vi "SW_Select_User.vi"() -> ()   [LabVIEW 2016]
uses:
  <vilib>/Utility/miscctls.llb/LVPointTypeDef.ctl
  <vilib>/Utility/config.llb/NI_LVConfig.lvlib
panel:
  out "TestComm indicator for Latching inside Events workaround":bool
  in  "Login tab":enum32{"Login", "Settings", "Manage users"}(tab)
  in  "Go to Tracker":bool
  in  "Select User":u16(ring) items=["Admin"]
  in  "Enter password":string
  in  "Jump to tracking":bool
  out "Comm. test results":bool
  in  "Test VISA Comms":bool
  in  "Save Settings":bool
  in  "VISA":refnum<visa-resource-name>="Tracker"
  in  "Cancel Users Update":bool
  in  "Save Users":bool
  in  "... or add new one":string
  in  "Reset or create password":string
  in  "Select User for update":u16(ring) items=["Researcher"]
  in  "Delete current user":bool
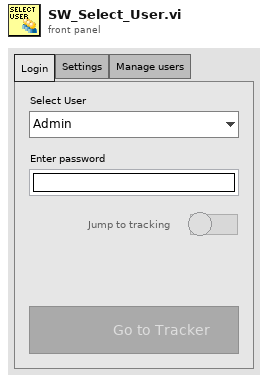
[diagram p1: front panel]
types:
  T1 = cluster{"Numeric Control":u32, "Numeric Control":u32}[]
  T2 = typedef "LVPointTypeDef.ctl" = cluster{"Horizontal":i16, "Vertical":i16}
  T3 = typedef "NI_LVConfig.lvlib/Config Data RefNum.ctl" = refnum<k1>
  T4 = typedef "eventvkey.ctl" = enum16{"ASCII", "Enter", "Return", "Shift", "Ctrl", "Alt", "Cmd", "Opt", "Caps", "NumLock", "Clear", "Break", "Up", "Down", "Left", "Right", "Insert", "Delete", "Home", "End", "PageUp", "PageDown", "Escape", "Help", "Pause", "ScrollLock", "F1", "F2", "F3", "F4", "F5", "F6", "F7", "F8", "F9", "F10", "F11", "F12", "F13", "F14", "F15", "F16", "F17", "F18", "F19", "F20", "F21", "F22", "F23", "F24", "Play", "VolumeUp", "VolumeDown", "Mute", "Two Byte Char"}
  T5 = enum32{"Page Enabled", "Page Disabled", "Page Disabled & Grayed"}
  T6 = enum8{"Enabled", "Disabled", "Disabled and Grayed Out"}
  T7 = cluster{"Data acquisition status":refnum<notifier>, "Play/Pause status":refnum<notifier>, "Recording status":refnum<notifier>}
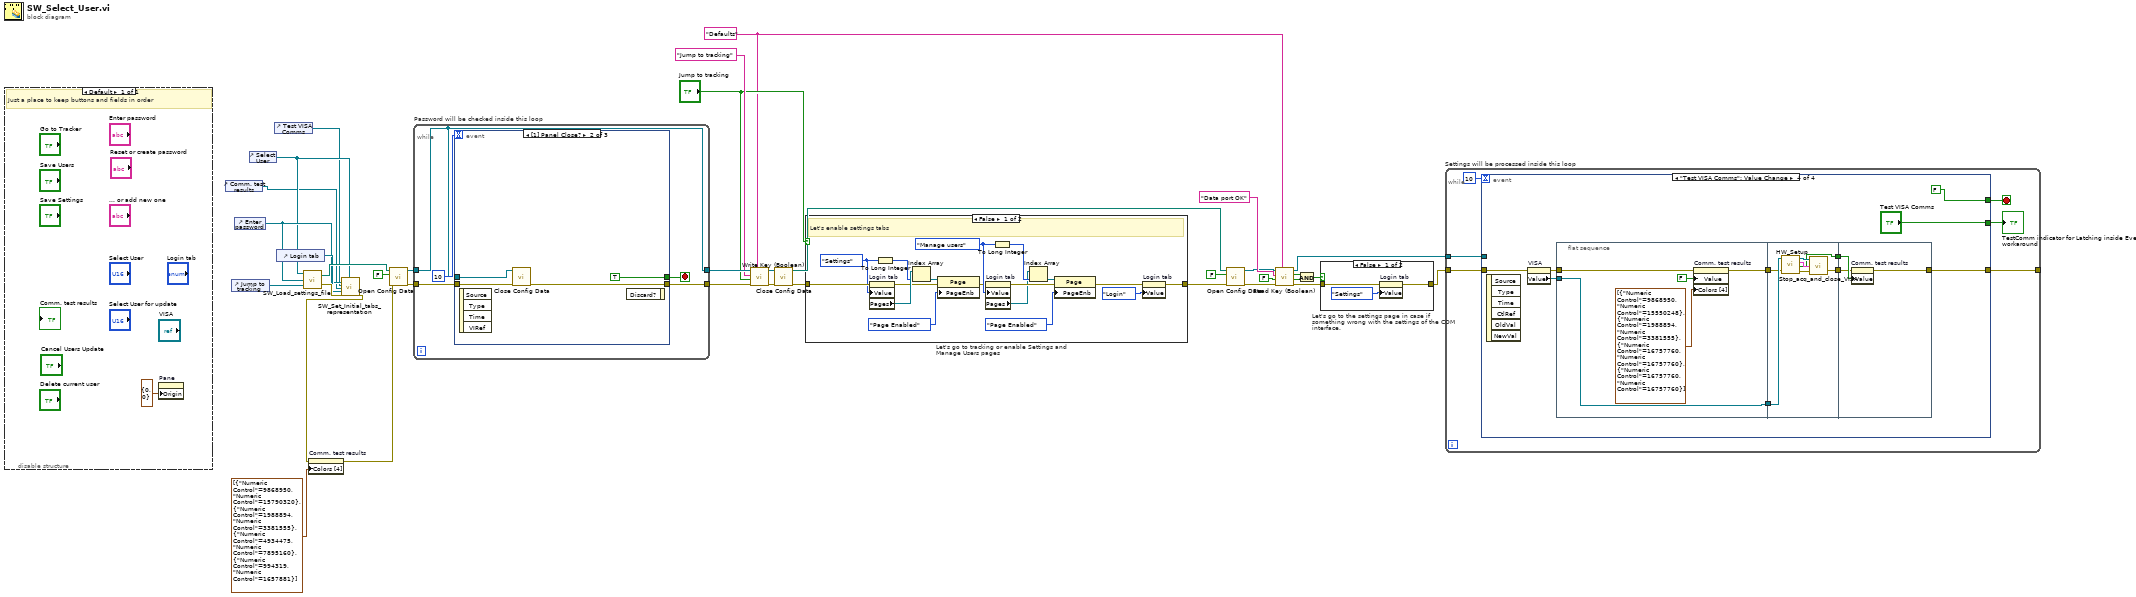
[diagram p0: block diagram]
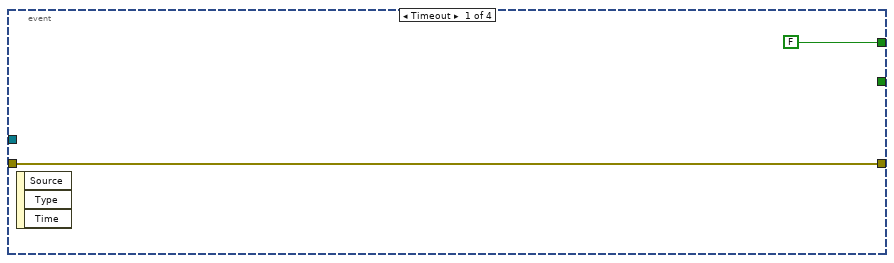
[diagram p2: hidden frame]
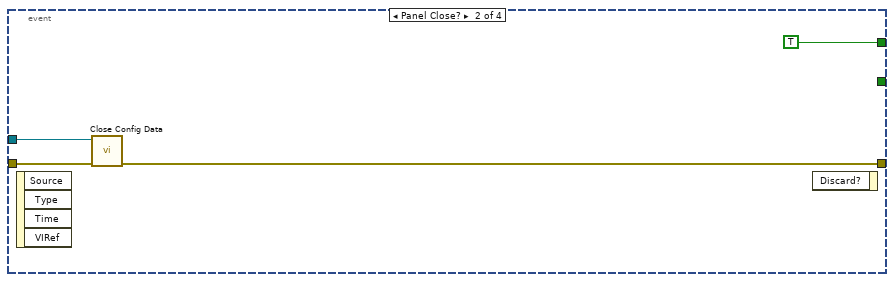
[diagram p3: hidden frame]
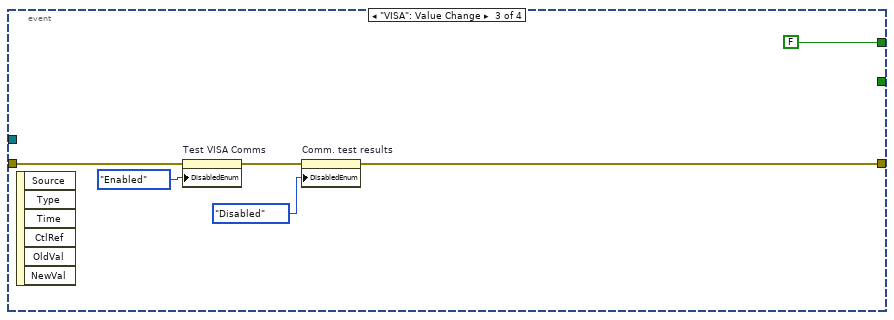
[diagram p4: hidden frame]
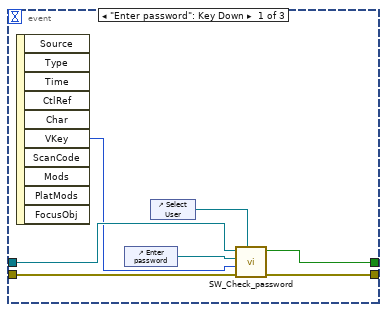
[diagram p7: hidden frame]
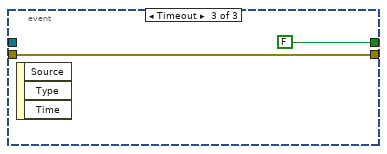
[diagram p8: hidden frame]
diagram:
  w26 = "Defaults" ("section")
  n1 = disable-structure shown="Default" {
    frame Enabled {
      # "Just a place to keep buttons and fields in order"
      n2 = property on="Pane" class="Pane"("Origin"=T2 {"Horizontal"=0, "Vertical"=0}) -> ()  [unwired: 2 in, 2 out]
    }
  }
  n3 = control-ref of="Comm. test results"() -> (w5:refnum<vi>)
  n4 = control-ref of="Jump to tracking"() -> (w35:refnum<vi>)
  n5 = control-ref of="Enter password"() -> (w9:refnum<vi>)
  n6 = control-ref of="Select User"() -> (w8:refnum<vi>)
  n7 = control-ref of="Test VISA Comms"() -> (w4:refnum<vi>)
  n8 = control-ref of="Login tab"() -> (w10:refnum<vi>)
  n9 = call "SW_Load_settings_file.vi"("Jump to tracking refnum in"=w35, "Password field reference in"=w9, "Researchers list reference in"=w8) -> ("error out"=w32:errorcluster, "Config file path"=w11:path)
  n10 = call "SW_Set_Initial_tabs_representation.vi"("Select User refnum in"=w8, "Enter password refnum in"=w9, "Test VISA Comms refnum in"=w4, "Comm. test results refnum in"=w5, "TabCtl Refnum in"=w10, "error in (no error)"=w32) -> ("error out"=w2:errorcluster)  [unwired: 13 in]
  n11 = property on="Comm. test results" class="Bool (strict)"(error in=w2, "Colors [4]"=T1 [{"Numeric Control"=9868950, "Numeric Control"=15790320}, {"Numeric Control"=1988894, "Numeric Control"=3381555}, {"Numeric Control"=4934475, "Numeric Control"=7895160}, {"Numeric Control"=994319, "Numeric Control"=1657881}]) -> (error out=w3:errorcluster)  [unwired: 1 in, 1 out]
  n12 = call <vilib>:"Open Config Data.vi"("error in (no error)"=w3, "create file if necessary (T)"=FALSE, "configuration file path"=w11) -> ("error out"=w33:errorcluster, "refnum"=w34:T3)  [unwired: 6 in, 1 out]
  n13 = while "Password will be checked inside this loop" {
    tunnel: w33 -> [w40]
    tunnel: w34 -> [w38]
    tunnel: [w39] -> w30
    tunnel: [w38] -> w31
    stop <- w37 stop-if-true
    n14 = event shown="[1] Panel Close?" {
      selector: _ -> [_ _ _]
      dyn-events: _ -> [_ _ _]
      timeout: 10 -> [_ _ _]
      tunnel: w40 -> [w48 w51 w53]
      tunnel: w38 -> [w47 w49 _]
      tunnel: [w45 TRUE ("Stop the loop") FALSE] -> w37
      tunnel: [w44 w50 w53] -> w39
      event "Enter password": Key Down {
        n15 = event-data() -> ("VKey"=w46:T4)  [unwired: 1 in, 9 out]
        n16 = control-ref of="Enter password"() -> (w42:refnum<vi>)
        n17 = control-ref of="Select User"() -> (w43:refnum<vi>)
        n18 = call "SW_Check_password.vi"("Ring Refnum"=w43, "error in (no error)"=w48, "Entered key"=w46, "Str Refnum"=w42, "Configuration file refnum in"=w47) -> ("error out"=w44:errorcluster, "Stop the loop"=w45:bool)  [unwired: 5 in]
      }
      event Panel Close? {
        n19 = event-data() -> ()  [unwired: 1 in, 4 out]
        n20 = call <vilib>:"Close Config Data.vi"("error in (no error)"=w51, "refnum"=w49) -> ("error out"=w50:errorcluster)  [unwired: 8 in, 1 out]
        n21 = event-data() -> ()  [unwired: 2 in, 1 out]
      }
      event Timeout {
        n22 = event-data() -> ()  [unwired: 1 in, 3 out]
      }
    }
  }
  n23 = call <vilib>:"Write Key (Boolean).vi"("section"=w26, "error in (no error)"=w30, "value"="Jump to tracking", "key"="Jump to tracking", "refnum"=w31) -> ("error out"=w20:errorcluster, "refnum out"=w18:T3)  [unwired: 4 in, 1 out]
  n24 = call <vilib>:"Close Config Data.vi"("error in (no error)"=w20, "refnum"=w18) -> ("error out"=w19:errorcluster, "file path"=w17:path)  [unwired: 8 in]
  n25 = case "Let's go to tracking or enable Settings and Manage Users pages" shown="False" "Jump to tracking" {
    tunnel: w19 -> [w71 w72]
    tunnel: [w56 w72] -> w16
    frame False {
      w60 = enum32{"Login", "Settings", "Manage users"}."Manage users" ("Login tab")
      w69 = enum32{"Login", "Settings", "Manage users"}."Settings" ("Login tab")
      # "Let's enable settings tabs"
      n26 = property on="Login tab" class="TabCtl (strict)"(error in=w71, "Value"=w69) -> (error out=w66:errorcluster, "Pages"=w70:refnum<vi>[])  [unwired: 1 in, 1 out]
      n27 = To Long Integer(number=w69) -> (32bit integer=w68:i32)
      n28 = Index Array(array=w70, index=w68) -> (element=w67:refnum<vi>)
      n29 = property class="Page"(reference=w67, error in=w66, "PageEnb"=T5."Page Enabled" ("Page Enabled State")) -> (error out=w58:errorcluster)  [unwired: 1 out]
      n30 = property on="Login tab" class="TabCtl (strict)"(error in=w58, "Value"=w60) -> (error out=w63:errorcluster, "Pages"=w59:refnum<vi>[])  [unwired: 1 in, 1 out]
      n31 = To Long Integer(number=w60) -> (32bit integer=w61:i32)
      n32 = Index Array(array=w59, index=w61) -> (element=w62:refnum<vi>)
      n33 = property class="Page"(reference=w62, error in=w63, "PageEnb"=T5."Page Enabled" ("Page Enabled State")) -> (error out=w57:errorcluster)  [unwired: 1 out]
      n34 = property on="Login tab" class="TabCtl (strict)"(error in=w57, "Value"=enum32{"Login", "Settings", "Manage users"}."Login" ("Login tab")) -> (error out=w56:errorcluster)  [unwired: 1 in, 1 out]
    }
    frame True {
      # "Here we'll check if everything else is OK and jump to tracking"
    }
  }
  n35 = call <vilib>:"Open Config Data.vi"("error in (no error)"=w16, "create file if necessary (T)"=FALSE, "configuration file path"=w17) -> ("error out"=w15:errorcluster, "refnum"=w14:T3)  [unwired: 6 in, 1 out]
  n36 = call <vilib>:"Read Key (Boolean).vi"("section"=w26, "error in (no error)"=w15, "default value"=FALSE, "key"="Data port OK", "refnum"=w14) -> ("error out"=w21:errorcluster, "value"=w23:bool, "found?"=w24:bool, "refnum out"=w6:T3)  [unwired: 3 in]
  n37 = And(x=w24, y=w23) -> (x .and. y?=w22:bool)
  n38 = case "Let's go to the settings page in case if something wrong with the settings of the COM interface." shown="False" w22 {
    tunnel: w21 -> [w73 w76]
    tunnel: [w75 w76] -> w7
    frame False {
      n39 = property on="Login tab" class="TabCtl (strict)"(error in=w73, "Value"=enum32{"Login", "Settings", "Manage users"}."Settings" ("Login tab")) -> (error out=w75:errorcluster)  [unwired: 1 in, 1 out]
    }
    frame True {
    }
  }
  n40 = while "Settings will be processed inside this loop" {
    tunnel: w7 -> [w80]
    tunnel: [w81] -> _
    tunnel: w6 -> [w78]
    stop <- w79 stop-if-true
    n41 = event shown="[3] \"Test VISA Comms\": Value Change" {
      selector: _ -> [_ _ _ _]
      dyn-events: _ -> [_ _ _ _]
      timeout: 10 -> [_ _ _ _]
      tunnel: [w84 w85 w90 w98] -> w81
      tunnel: w80 -> [w84 w86 w94 w103]
      tunnel: [FALSE TRUE FALSE FALSE] -> w79
      tunnel: w78 -> [_ w87 _ _]
      tunnel: [_ _ _ "Test VISA Comms"] -> w77
      event Timeout {
        n42 = event-data() -> ()  [unwired: 1 in, 3 out]
      }
      event Panel Close? {
        n43 = event-data() -> ()  [unwired: 1 in, 4 out]
        n44 = call <vilib>:"Close Config Data.vi"("error in (no error)"=w86, "refnum"=w87) -> ("error out"=w85:errorcluster)  [unwired: 8 in, 1 out]
        n45 = event-data() -> ()  [unwired: 2 in, 1 out]
      }
      event "VISA": Value Change {
        n46 = event-data() -> ()  [unwired: 1 in, 6 out]
        n47 = property on="Test VISA Comms" class="Bool"(error in=w94, "DisabledEnum"=T6."Enabled" ("Disabled")) -> (error out=w93:errorcluster)  [unwired: 1 in, 1 out]
        n48 = property on="Comm. test results" class="Bool (strict)"(error in=w93, "DisabledEnum"=T6."Disabled" ("Disabled")) -> (error out=w90:errorcluster)  [unwired: 1 in, 1 out]
      }
      event "Test VISA Comms": Value Change {
        n49 = event-data() -> ()  [unwired: 1 in, 6 out]
        n50 = property on="VISA" class="VISAName"(error in=w103) -> (error out=w102:errorcluster, "Value"=w101:refnum<visa-resource-name>)  [unwired: 1 in, 1 out]
        n51 = flat-sequence {
          tunnel: w102 -> [w107]
          tunnel: w101 -> [w109]
          tunnel: [w109] -> w100
          tunnel: [w106] -> w99
          tunnel: w100 -> [w116]
          tunnel: w99 -> [w111]
          tunnel: [w112] -> w96
          tunnel: [w110] -> w95
          tunnel: [w119] -> w98
          tunnel: w95 -> [w117]
          tunnel: w96 -> [w118]
          frame #0 {
            n52 = property on="Comm. test results" class="Bool (strict)"(error in=w107, "Value"=FALSE ("Comm. test results"), "Colors [4]"=T1 [{"Numeric Control"=9868950, "Numeric Control"=15550248}, {"Numeric Control"=1988894, "Numeric Control"=3381555}, {"Numeric Control"=16757760, "Numeric Control"=16757760}, {"Numeric Control"=16757760, "Numeric Control"=16757760}]) -> (error out=w106:errorcluster)  [unwired: 1 in, 1 out]
          }
          frame #1 {
            n53 = call "HW_Setup.vi"("VISA resource name in"=w116, "error in"=w111) -> ("VISA resource name out"=w115:refnum<visa-resource-name>, "Data flow controls"=w114:T7, "Instrument OK?"=w112:bool, "error out"=w113:errorcluster)  [unwired: 1 in]
            n54 = call "Stop_acq_and_close_VISA.vi"("error in"=w113, "Data flow controls in"=w114, "VISA resource name in"=w115) -> ("error out"=w110:errorcluster)  [unwired: 1 out]
          }
          frame #2 {
            n55 = property on="Comm. test results" class="Bool (strict)"(error in=w117, "Value"=w118) -> (error out=w119:errorcluster)  [unwired: 1 in, 1 out]
          }
        }
      }
    }
    "TestComm indicator for Latching inside Events workaround" <- w77
  }
